vi "Generate Effect Images.vi"(10 "Effect Types":string[](array[string]), 11 "Path":path) -> (3 "Effect Images":variant)   [LabVIEW 2019]
doc: "Generates arrays of Effect Images and Small Effect Images and associates each image with an Effect Name from the City Card list."
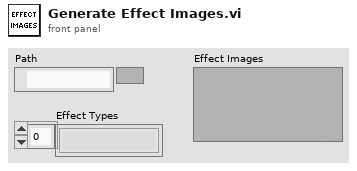
[diagram p1: front panel]
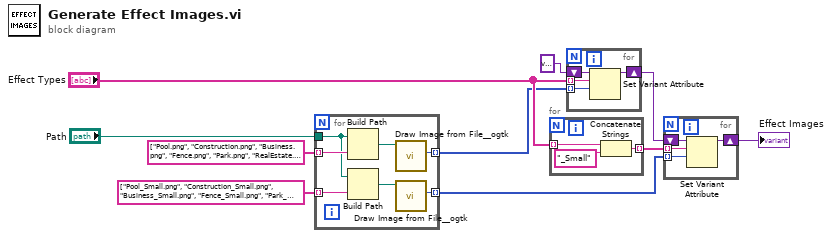
[diagram p0: block diagram]
diagram:
  n1 = for {
    tunnel: [w16] -> w4 mode=indexing
    tunnel: "Path" -> [w13]
    tunnel: string[] ["Pool.png", "Construction.png", "Business.png", "Fence.png", "Park.png", "RealEstate.png"] ("name or relative path") -> [w15] mode=indexing
    tunnel: string[] ["Pool_Small.png", "Construction_Small.png", "Business_Small.png", "Fence_Small.png", "Park_Small.png", "RealEstate_Small.png"] ("name or relative path") -> [w12] mode=indexing
    tunnel: [w11] -> w7 mode=indexing
    n2 = Build Path(base path=w13, name or relative path=w15) -> (appended path=w17:path)
    n3 = Build Path(base path=w13, name or relative path=w12) -> (appended path=w14:path)
    n4 = call <userlib>:"Draw Image from File__ogtk.vi"("path to image file"=w17) -> ("new picture"=w16:picture)  [unwired: 7 in, 3 out]
    n5 = call <userlib>:"Draw Image from File__ogtk.vi"("path to image file"=w14) -> ("new picture"=w11:picture)  [unwired: 7 in, 3 out]
  }
  n6 = for {
    tunnel: "Effect Types" -> [w19] mode=indexing
    tunnel: [w18] -> w9 mode=indexing
    n7 = Concatenate Strings(w19, "_Small" ("string")) -> (w18:string)
  }
  n8 = for {
    tunnel: "Effect Types" -> [w24] mode=indexing
    tunnel: w4 -> [w23] mode=indexing
    shift-right: [w22] -> w5
    shift-left: variant -> [w21]
    n9 = Set Variant Attribute(Variant=w21, name=w24, value=w23) -> (Variant out=w22:variant)  [unwired: 1 in, 2 out]
  }
  n10 = for {
    tunnel: w7 -> [w28] mode=indexing
    shift-right: [w27] -> w6
    shift-left: w5 -> [w26]
    tunnel: w9 -> [w25] mode=indexing
    n11 = Set Variant Attribute(Variant=w26, name=w25, value=w28) -> (Variant out=w27:variant)  [unwired: 1 in, 2 out]
  }
  "Effect Images" <- w6
